vi "GV_YscaleAdd.vi"(8 "error in (no error)":errorcluster, 9 "Coords":T1, 11 "Gviewer in":refnum<class "Gviewer.lvclass">) -> (0 "error out":errorcluster, 3 "Gviewer out":refnum<class "Gviewer.lvclass">)   [LabVIEW 2020, in "Sgraph_lib_V1.lvlib" / "Gviewer.lvclass"]
doc: "Add an Yscale when selected on mouse click"
uses:
  Gviewer.lvclass
  <vilib>/Utility/miscctls.llb/LVPoint32TypeDef.ctl
  Gviewer.lvclass/Gviewer.ctl
  controls/YgraphDef.ctl
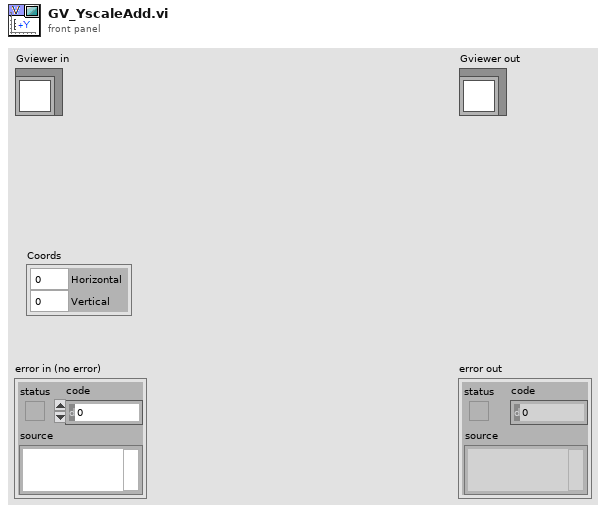
[diagram p1: front panel]
types:
  T1 = typedef "LVPoint32TypeDef.ctl" = cluster{"Horizontal":i32, "Vertical":i32}
  T2 = typedef "Sgraph_lib_V1.lvlib/Gviewer.lvclass/YgraphDef.ctl" = cluster{"Plot":i32, "X(%)":dbl}
  T3 = typedef "LVRectTypeDef.ctl" = cluster{"Left":i16, "Top":i16, "Right":i16, "Bottom":i16}
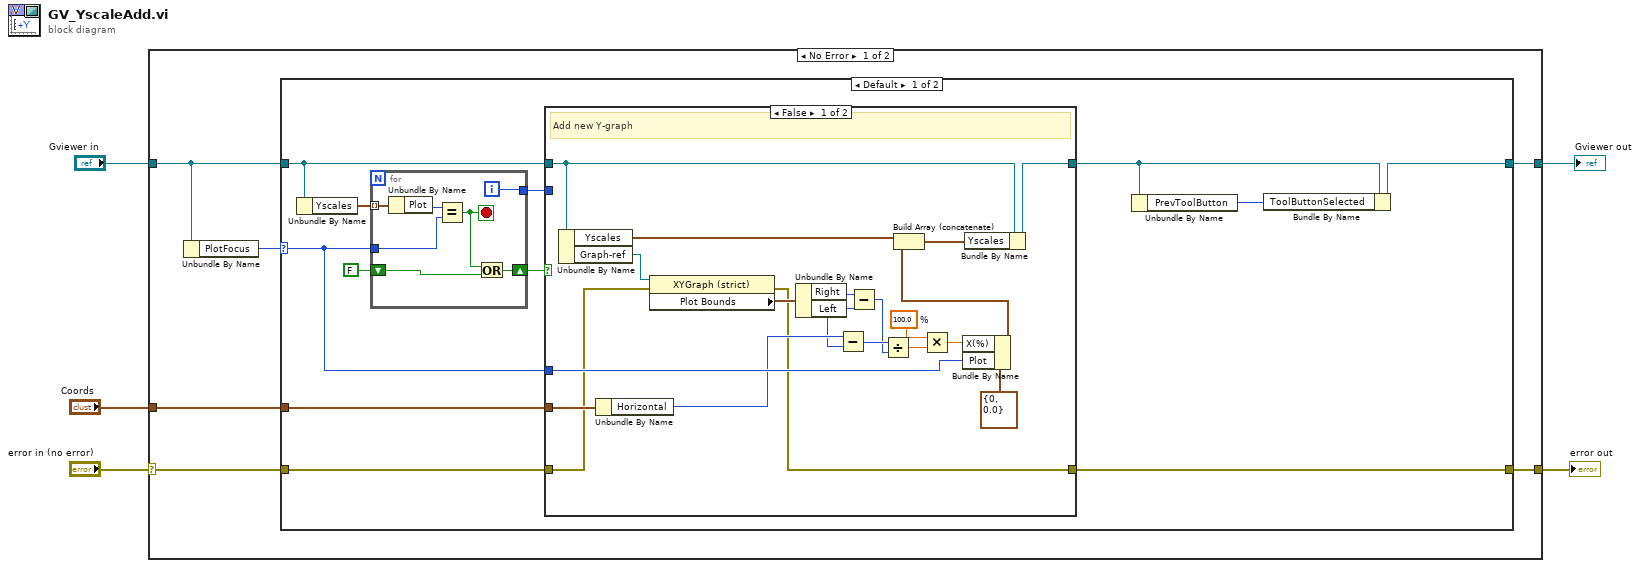
[diagram p0: block diagram]
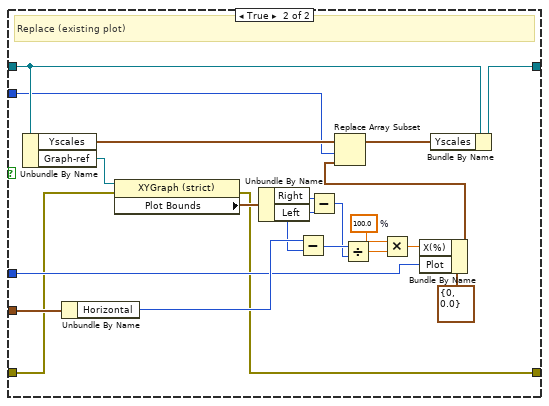
[diagram p2: hidden frame]
diagram:
  n1 = case shown="No Error" "error in (no error)" {
    selector: "error in (no error)" -> [w7 w75]
    tunnel: [w6 w75] -> w4
    tunnel: [w11 w74] -> w2
    tunnel: "Gviewer in" -> [w10 w74]
    tunnel: "Coords" -> [w8 _]
    frame No Error {
      n2 = Unbundle By Name(w10) -> ("PlotFocus"=w9:i32)
      n3 = case shown="Default" w9 {
        selector: w9 -> [w17 _]
        tunnel: w10 -> [w20 w73]
        tunnel: w7 -> [w19 w72]
        tunnel: [w12 w73] -> w11
        tunnel: [w18 w72] -> w6
        tunnel: w8 -> [w16 _]
        frame Default {
          n4 = Unbundle By Name(w20) -> ("Yscales"=w23:T2[])
          n5 = for {
            tunnel: w23 -> [w71] mode=indexing
            tunnel: w17 -> [w69]
            shift-right: [w66] -> w21
            shift-left: FALSE -> [w67]
            tunnel: [w65] -> w15
            i -> [w65]
            stop <- w68 stop-if-true
            n6 = Unbundle By Name(w71) -> ("Plot"=w70:i32)
            n7 = Equal?(x=w70, y=w69) -> (x = y?=w68:bool)
            n8 = Or(x=w68, y=w67) -> (x .or. y?=w66:bool)
          }
          n9 = case shown="False" w21 {
            tunnel: w20 -> [w37 w48]
            tunnel: w19 -> [w25 w51]
            tunnel: [w38 w47] -> w13
            tunnel: [w24 w44] -> w18
            tunnel: w17 -> [w41 w53]
            tunnel: w16 -> [w33 w52]
            tunnel: w15 -> [_ w45]
            frame False {
              w27 = 100.0  # %
              # "Add new Y-graph"
              n10 = Unbundle By Name(w37) -> ("Yscales"=w43:T2[], "Graph-ref"=w34:refnum<vi>)
              n11 = Unbundle By Name(w33) -> ("Horizontal"=w36:i32)
              n12 = property class="XYGraph (strict)"(reference=w34, error in=w25) -> (error out=w24:errorcluster, "Plot Bounds"=w35:T3)  [unwired: 1 out]
              n13 = Unbundle By Name(w35) -> ("Right"=w32:i16, "Left"=w31:i16)
              n14 = Subtract(x=w36, y=w31) -> (x-y=w30:i32)
              n15 = Subtract(x=w32, y=w31) -> (x-y=w29:i16)
              n16 = Divide(x=w30, y=w29) -> (x/y=w28:dbl)
              n17 = Multiply(x=w27, y=w28) -> (x*y=w26:dbl)
              n18 = Bundle By Name(cluster=T2 {"Plot"=0, "X(%)"=0.0} ("Ygraph"), "X(%)"=w26, "Plot"=w41) -> (w40:T2)
              n19 = Build Array (concatenate)(w43, w40) -> (w39:T2[])
              n20 = Bundle By Name(cluster=w37, "Yscales"=w39) -> (w38:refnum<class "Gviewer.lvclass">)
            }
            frame True {
              w55 = 100.0  # %
              # "Replace (existing plot)"
              n21 = Unbundle By Name(w48) -> ("Yscales"=w50:T2[], "Graph-ref"=w62:refnum<vi>)
              n22 = Unbundle By Name(w52) -> ("Horizontal"=w64:i32)
              n23 = property class="XYGraph (strict)"(reference=w62, error in=w51) -> (error out=w44:errorcluster, "Plot Bounds"=w63:T3)  [unwired: 1 out]
              n24 = Unbundle By Name(w63) -> ("Right"=w61:i16, "Left"=w60:i16)
              n25 = Subtract(x=w64, y=w60) -> (x-y=w59:i32)
              n26 = Subtract(x=w61, y=w60) -> (x-y=w58:i16)
              n27 = Divide(x=w59, y=w58) -> (x/y=w57:dbl)
              n28 = Multiply(x=w55, y=w57) -> (x*y=w56:dbl)
              n29 = Bundle By Name(cluster=T2 {"Plot"=0, "X(%)"=0.0} ("Ygraph"), "X(%)"=w56, "Plot"=w53) -> (w46:T2)
              n30 = Replace Array Subset(array=w50, new element=w46, index=w45) -> (w49:T2[])
              n31 = Bundle By Name(cluster=w48, "Yscales"=w49) -> (w47:refnum<class "Gviewer.lvclass">)
            }
          }
          n32 = Unbundle By Name(w13) -> ("PrevToolButton"=w14:i32)
          n33 = Bundle By Name(cluster=w13, "ToolButtonSelected"=w14) -> (w12:refnum<class "Gviewer.lvclass">)
        }
        frame -1 {
        }
      }
    }
    frame Error {
    }
  }
  "error out" <- w4
  "Gviewer out" <- w2
